vi "VerifyArguments.vi"(8 "error in (no error)":errorcluster, 11 "DiffVI in":refnum<class "DiffVI.lvclass">) -> (0 "error out":errorcluster, 3 "DiffVI out":refnum<class "DiffVI.lvclass">)   [LabVIEW 2020, in "DiffVI.lvclass"]
uses:
  DiffVI.lvclass
  Program Files (x86)/National Instruments/Shared/LabVIEW CLI/Operations/Utilities/OperationErrorType.ctl
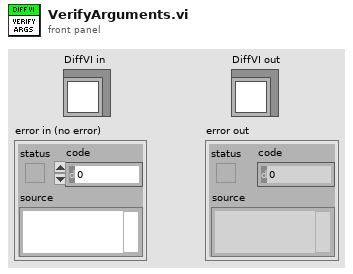
[diagram p1: front panel]
types:
  T1 = typedef "OperationErrorType.ctl" = enum16{"RequiredArgumentMissing", "UnknownArguments", "LoggerSetMultipleTimes", "OperationBrokenError"}
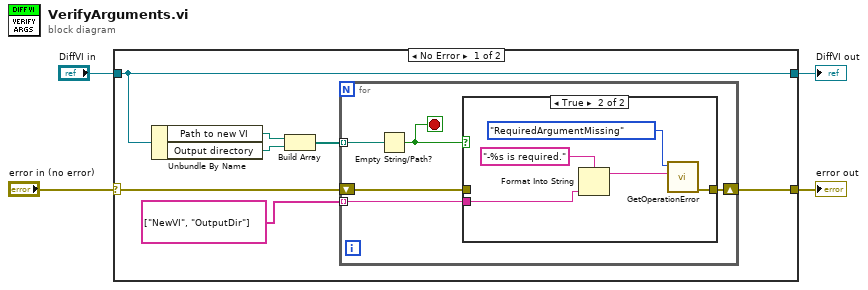
[diagram p0: block diagram]
diagram:
  n1 = case shown="No Error" "error in (no error)" {
    selector: "error in (no error)" -> [w11 w24]
    tunnel: [w10 w24] -> w2
    tunnel: [w9 w23] -> w3
    tunnel: "DiffVI in" -> [w9 w23]
    frame No Error {
      n2 = Unbundle By Name(w9) -> ("Path to new VI"=w7:path, "Output directory"=w6:path)
      n3 = Build Array(w7, w6) -> (w5:path[])
      n4 = for {
        shift-right: [w15] -> w10
        shift-left: w11 -> [w16]
        tunnel: string[] ["NewVI", "OutputDir"] ("Additional Information") -> [w14] mode=indexing
        tunnel: w5 -> [w13] mode=indexing
        stop <- w12 stop-if-true
        n5 = Empty String/Path?(string/path=w13) -> (empty?=w12:bool)
        n6 = case shown="True" w12 {
          tunnel: w16 -> [w17 _]
          tunnel: [w17 w22] -> w15
          tunnel: w14 -> [_ w18]
          frame False {
          }
          frame True {
            n7 = Format Into String(format string="-%s is required.", w18) -> (resulting string=w19:string)  [unwired: 2 in, 1 out]
            n8 = call "GetOperationError.vi"("Additional Information"=w19, "Operation Error Type"=OperationErrorType."RequiredArgumentMissing") -> ("error out"=w22:errorcluster)  [unwired: 9 in]
          }
        }
      }
    }
    frame Error {
    }
  }
  "DiffVI out" <- w3
  "error out" <- w2
